vi "打断循环.vi"() -> ()   [LabVIEW 2018]
panel:
  in  "停止":bool
  out "数值":i32
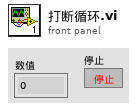
[diagram p1: front panel]
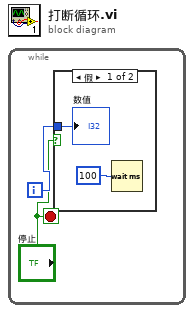
[diagram p0: block diagram]
diagram:
  n1 = while {
    i -> [w2]
    stop <- "停止" stop-if-true
    n2 = case shown="假" "停止" {
      tunnel: w2 -> [w3 _]
      frame False {
        n3 = Wait (ms)(milliseconds to wait=u32 100 ("等待时间（毫秒）")) -> ()  [unwired: 1 out]
        "数值" <- w3
      }
      frame True {
      }
    }
  }
